vi "To Array U16 2D.vi"(8 "error in":errorcluster, 11 "Generic Image in":refnum<class "Generic Image.lvclass">) -> (0 "error out":errorcluster, 1 "Timestamp":timestamp, 2 "U16":u16[][](array[numeric]))   [LabVIEW 2025, in "Generic Image.lvclass"]
uses:
  Generic Image.lvclass
  Generic Image.lvclass/Generic Image.ctl
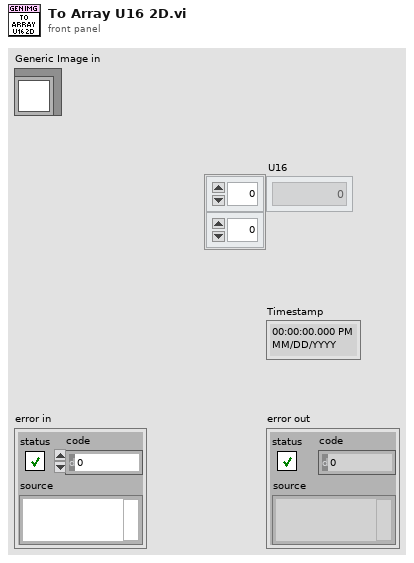
[diagram p1: front panel]
types:
  T1 = typedef "Generic Image.lvclass/Pixel Format.ctl" = enum16{"Grayscale (U8)", "Grayscale (I16)", "Grayscale (SGL)", "Complex (CSG)", "RGB (U32)", "HSL (U32)", "RGB (U64)", "Grayscale (U16)"}
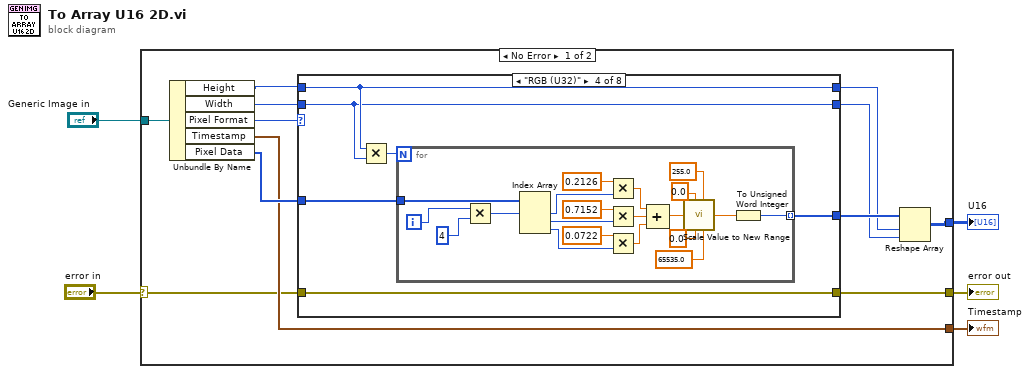
[diagram p0: block diagram]
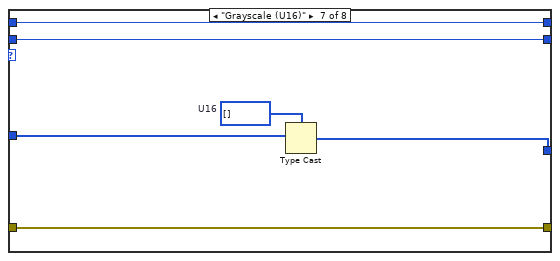
[diagram p7: hidden frame]
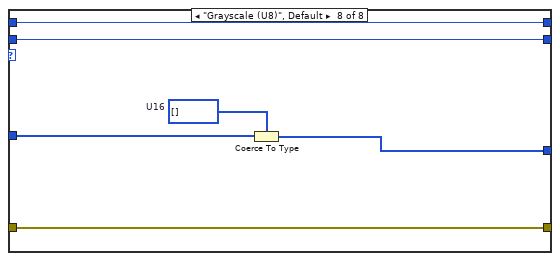
[diagram p8: hidden frame]
diagram:
  n1 = case shown="No Error" "error in" {
    selector: "error in" -> [w14 w76]
    tunnel: "Generic Image in" -> [w6 _]
    tunnel: [w15 _] -> w5
    tunnel: [w13 w76] -> w3
    tunnel: [w11 _] -> w2
    frame No Error {
      n2 = Unbundle By Name(w6) -> ("Height"=w10:i32, "Width"=w9:i32, "Pixel Format"=w16:T1, "Timestamp"=w15:timestamp, "Pixel Data"=w17:u8[])
      n3 = case shown="\"RGB (U32)\"" w16 {
        tunnel: w17 -> [w20 w24 w28 w34 w58 w62 w69 w75]
        tunnel: w14 -> [w21 w25 w29 w35 w59 w63 w66 w72]
        tunnel: [w21 w25 w29 w35 w59 w63 w66 w72] -> w13
        tunnel: [w20 w24 w28 w32 w58 w62 w67 w73] -> w12
        tunnel: w10 -> [w19 w23 w27 w31 w57 w61 w65 w71]
        tunnel: w9 -> [w18 w22 w26 w30 w56 w60 w64 w70]
        tunnel: [w19 w23 w27 w31 w57 w61 w65 w71] -> w8
        tunnel: [w18 w22 w26 w30 w56 w60 w64 w70] -> w7
        frame "Grayscale (I16)" {
        }
        frame "Grayscale (SGL)" {
        }
        frame "Complex (CSG)" {
        }
        frame "RGB (U32)" {
          n4 = Multiply(x=w31, y=w30) -> (x*y=w33:i32)
          n5 = for {
            N: w33 -> [_]
            tunnel: w34 -> [w55]
            tunnel: [w38] -> w32 mode=indexing
            i -> [w54]
            n6 = Multiply(x=w54, y=4 ("x")) -> (x*y=w43:i32)
            n7 = Index Array(array=w55, index #1=w43) -> (element #1=w52:u8, element #2=w50:u8, element #3=w47:u8)  [unwired: 2 in]
            n8 = Multiply(x=0.2126, y=w52) -> (x*y=w44:dbl)
            n9 = Multiply(x=0.7152, y=w50) -> (x*y=w45:dbl)
            n10 = Multiply(x=0.0722, y=w47) -> (x*y=w46:dbl)
            n11 = Compound Arithmetic op=ADD(w44, w45, w46) -> (w42:dbl)
            n12 = call <vilib>:"Scale Value to New Range.vi"("original minimum"=0.0, "original value"=w42, "new minimum"=0.0, "original maximum"=255.0, "new maximum"=65535.0) -> ("scaled value"=w39:dbl)  [unwired: 4 in]
            n13 = To Unsigned Word Integer(number=w39) -> (unsigned 16bit integer=w38:u16)
          }
        }
        frame "HSL (U32)" {
        }
        frame "RGB (U64)" {
        }
        frame "Grayscale (U16)" {
          w68 = u16[] []  # U16
          n14 = Type Cast(type=w68, x=w69) -> (*(type *) &x=w67:u16[])
        }
        frame "Grayscale (U8)", Default {
          w74 = u16[] []  # U16
          n15 = Coerce To Type(0:w75, 1:w74) -> (2:w73:u16[])
        }
      }
      n16 = Reshape Array(w12, w8, w7) -> (w11:u16[][])
    }
    frame Error {
    }
  }
  "error out" <- w3
  "U16" <- w2
  "Timestamp" <- w5
